vi "NIVisOpenCV AprilTagdetection.vi"(5 "refine Edges":bool=TRUE, 6 "threads":i32=2, 7 "blur":dbl step=0.1, 8 "error in":errorcluster, 9 "decimate":dbl=2.0, 10 "Tag Familys":string[](array[combo])=["16h5"], 11 "Image Src":T2) -> (0 "error out":errorcluster, 1 "Execution Time":dbl, 2 "Detected Tags":T1(array[cluster]), 3 "Image Dst Out":T2)   [LabVIEW 2025]
doc: "<b> NIVisOpenCV April Tag Detection</b> searches the image and describes tags in the Tag Familys. Parameters can be used to improve performance."
uses:
  <vilib>/vision/Image Controls.llb/IMAQ Image.ctl
  FRC_OpenCVExtensions.dll
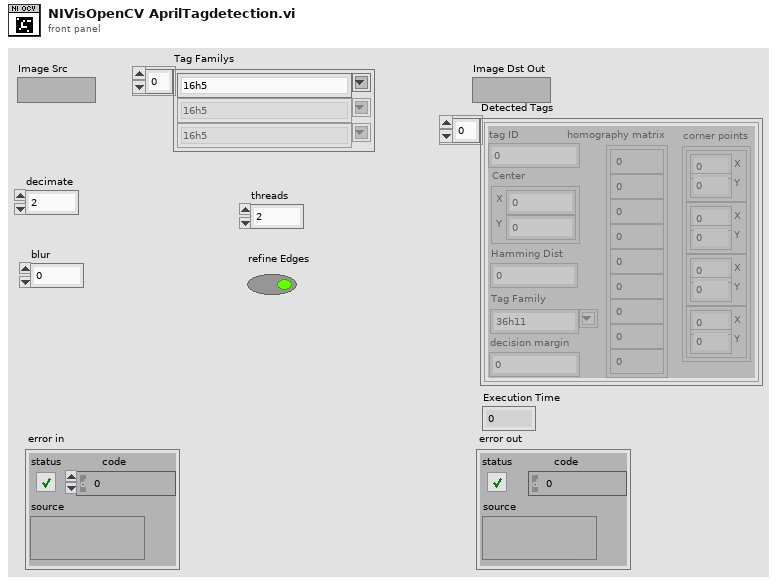
[diagram p1: front panel]
types:
  T1 = cluster{"tag ID":i32, "Center":cluster{"X":dbl, "Y":dbl}, "homography matrix":dbl[], "decision margin":dbl, "Hamming Dist":i32, "corner points":cluster{"X":dbl, "Y":dbl}[], "Tag Family":string}[]
  T2 = typedef "IMAQ Image.ctl" = refnum<image>
  T3 = cluster{"tag ID":i32, "Center":cluster{"X":dbl, "Y":dbl}, "Homography Matrix":dbl[], "dec margin":dbl, "Hamming Dist":i32, "Corner Points":cluster{"X":dbl, "Y":dbl}[], "familyID":i32}[]
  T4 = cluster{"tag ID":i32, "Center":cluster{"X":dbl, "Y":dbl}, "Homography Matrix":dbl[], "dec margin":dbl, "Hamming Dist":i32, "Corner Points":cluster{"X":dbl, "Y":dbl}[], "Tag Family":string}
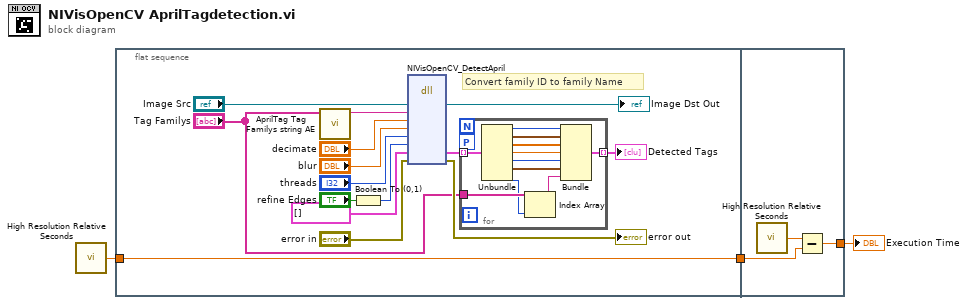
[diagram p0: block diagram]
diagram:
  n1 = call <vilib>:"High Resolution Relative Seconds.vi"() -> ("relative seconds"=w3:dbl)
  n2 = flat-sequence {
    tunnel: w3 -> [w4]
    tunnel: [w4] -> w2
    tunnel: w2 -> [w31]
    tunnel: [w30] -> w1
    frame #0 {
      # "Convert family ID to family Name"
      n3 = call "AprilTag Tag Familys string AE.vi"("Tag Familys"="Tag Familys") -> ("Tag Familys String"=w5:string)  [unwired: 10 in]
      n4 = Boolean To (0,1)(Boolean="refine Edges") -> (0, 1=w8:i16)
      n5 = dll-call lib="FRC_OpenCVExtensions.*" fn="NIVisOpenCV_DetectApril"("ImageA"="Image Src", "famName"=w5, "decimationValue"="decimate", "blurValue"="blur", "workerThreads"="threads", "refineEdges"=w8, "ImageAPoints"=T3 [] ("Detected Tags"), "error"="error in") -> ("ImageA"=→"Image Dst Out":T2, "ImageAPoints"=w6:T3, "error"=→"error out":errorcluster)  [unwired: 9 in, 2 out]
      n6 = for {
        tunnel: w6 -> [w29] mode=indexing
        tunnel: "Tag Familys" -> [w22]
        tunnel: [w19] -> w10 mode=indexing
        workers-P: _ -> [_]
        n7 = Unbundle(w29) -> ("tag ID"=w28:i32, "Center"=w27:cluster{"X":dbl, "Y":dbl}, "Homography Matrix"=w26:dbl[], "dec margin"=w25:dbl, "Hamming Dist"=w24:i32, "Corner Points"=w23:cluster{"X":dbl, "Y":dbl}[], "familyID"=w21:i32)
        n8 = Index Array(array=w22, index=w21) -> (element=w20:string)
        n9 = Bundle("tag ID"=w28, "Center"=w27, "Homography Matrix"=w26, "dec margin"=w25, "Hamming Dist"=w24, "Corner Points"=w23, "Tag Family"=w20) -> (w19:T4)  [unwired: 1 in]
      }
      "Detected Tags" <- w10
    }
    frame #1 {
      n10 = call <vilib>:"High Resolution Relative Seconds.vi"() -> ("relative seconds"=w32:dbl)
      n11 = Subtract(x=w32, y=w31) -> (x-y=w30:dbl)
    }
  }
  "Execution Time" <- w1
